vi "OutputRF.vi"(6 "Route Names":string[](array[string]), 7 "output enabled":bool=TRUE, 8 "error in (no error)":errorcluster, 9 "Power (dBm)":dbl, 10 "Frequency (Hz)":dbl, 11 "SigGen_MXG in":refnum<class "SigGen_MXG.lvclass">) -> (0 "error out":errorcluster, 3 "SigGen_MXG out":refnum<class "SigGen_MXG.lvclass">)   [LabVIEW 2014, in "SigGen_MXG.lvclass"]
uses:
  SigGen_MXG.lvclass
  SigGen_MXG.lvclass/SigGen_MXG.ctl
  data/Agilent PSG MXG Series.lvlib
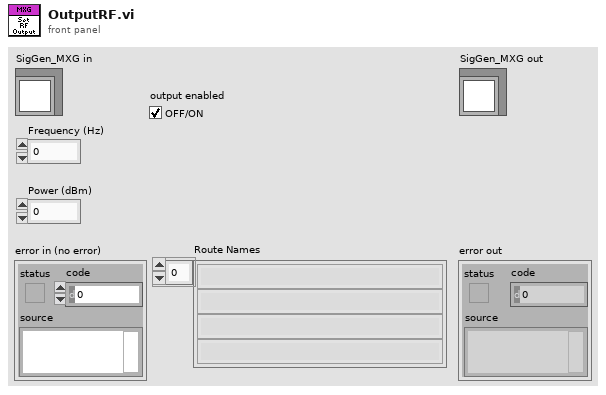
[diagram p1: front panel]
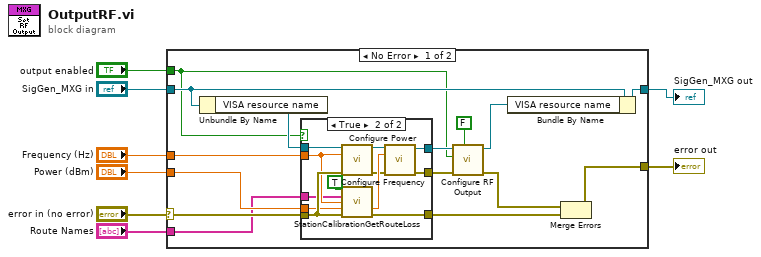
[diagram p0: block diagram]
diagram:
  n1 = case shown="No Error" "error in (no error)" {
    selector: "error in (no error)" -> [w21 w38]
    tunnel: "SigGen_MXG in" -> [w15 w39]
    tunnel: [w16 w38] -> w7
    tunnel: [w14 w39] -> w5
    tunnel: "output enabled" -> [w9 _]
    tunnel: "Frequency (Hz)" -> [w12 _]
    tunnel: "Power (dBm)" -> [w11 _]
    tunnel: "Route Names" -> [w10 _]
    frame No Error {
      n2 = Unbundle By Name(w15) -> ("VISA resource name"=w23:refnum<visa-resource-name>)
      n3 = case shown="True" w9 {
        tunnel: w23 -> [w25 w37]
        tunnel: w21 -> [w24 w36]
        tunnel: [w24 w35] -> w20
        tunnel: [w25 w31] -> w19
        tunnel: [w24 w30] -> w18
        tunnel: w12 -> [_ w29]
        tunnel: w11 -> [_ w28]
        tunnel: w10 -> [_ w27]
        frame False {
        }
        frame True {
          n4 = call "Configure Frequency.vi"("VISA resource name"=w37, "Frequency (100 kHz)"=w29, "error in (no error)"=w36) -> ("VISA resource name out"=w33:refnum<visa-resource-name>, "error out"=w32:errorcluster)  [unwired: 6 in, 5 out]
          n5 = call "StationCalibrationGetRouteLoss.vi"("Calibration Enabled"=TRUE, "Route Names"=w27, "Frequency"=w29, "Power Level"=w28, "error in (no error)"=w36) -> ("Adjusted Power Level"=w34:dbl, "error out"=w35:errorcluster)  [unwired: 7 in, 2 out]
          n6 = call "Configure Power.vi"("VISA resource name"=w33, "Power (-130 dBm)"=w34, "error in (no error)"=w32) -> ("VISA resource name out"=w31:refnum<visa-resource-name>, "error out"=w30:errorcluster)  [unwired: 7 in, 4 out]
        }
      }
      n7 = call "Configure RF Output.vi"("Enable Modulation (T:Enable)"=FALSE, "error in (no error)"=w18, "Enable RF Output (F:Disable)"=w9, "VISA resource name"=w19) -> ("error out"=w17:errorcluster, "VISA resource name out"=w13:refnum<visa-resource-name>)  [unwired: 4 in, 2 out]
      n8 = Bundle By Name(cluster=w15, "VISA resource name"=w13) -> (w14:refnum<class "SigGen_MXG.lvclass">)
      n9 = Merge Errors(w17, w20) -> (w16:errorcluster)
    }
    frame Error {
    }
  }
  "error out" <- w7
  "SigGen_MXG out" <- w5
